vi "Change Macro Name in Listbox.vi"(9 "Call Data":variant, 10 "Popup Value":variant, 11 "Macros List in":cluster{"enabled?":bool, "macro name":string}[](array[cluster])) -> (3 "Macros List out":cluster{"enabled?":bool, "macro name":string}[](array[cluster]))   [LabVIEW 2016, in "Hardware.lvlib" / "Motions.lvlib" / "Motions Configuration.lvclass"]
uses:
  <userlib>/Common Components/Hardware/Abstract System/Motions/Motions Config/Motions Configuration.lvclass
  <userlib>/TSPopup/TSPopup.Grid.Cell Info.ctl
  <userlib>/TSPopup/TSPopup.Data Type.ctl
  <userlib>/TSPopup/TSPopup.lvclass
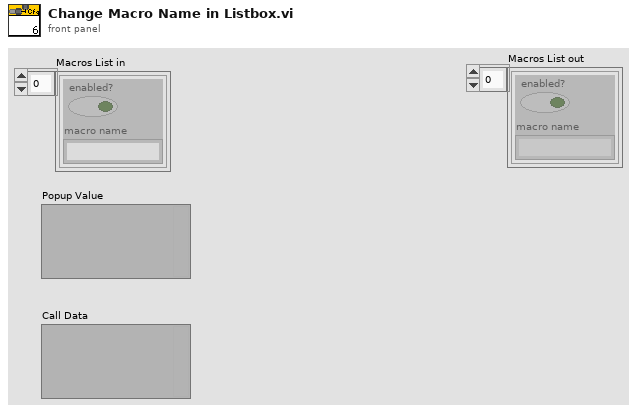
[diagram p1: front panel]
types:
  T1 = typedef "TSPopup.lvlib/TSPopup.lvclass/TSPopup.Grid.Cell Info.ctl" = cluster{"Tag":string, "Row":i32, "Column":i32, "In Symbol?":bool, "In Data?":bool, "Cell String":string, "Ctl Refnum":refnum<vi>, "Prop Type":T2, "Ring Strings":string[]}
  T2 = typedef "TSPopup.lvlib/TSPopup.lvclass/TSPopup.Data Type.ctl" = enum16{"Unkown", "NO POPUP", "String", "Integer", "Float", "Color", "Boolean", "Ring", "Captioned String", "Captioned Integer", "Button Color", "2 Int Cluster", "4 Int Cluster", "check"}
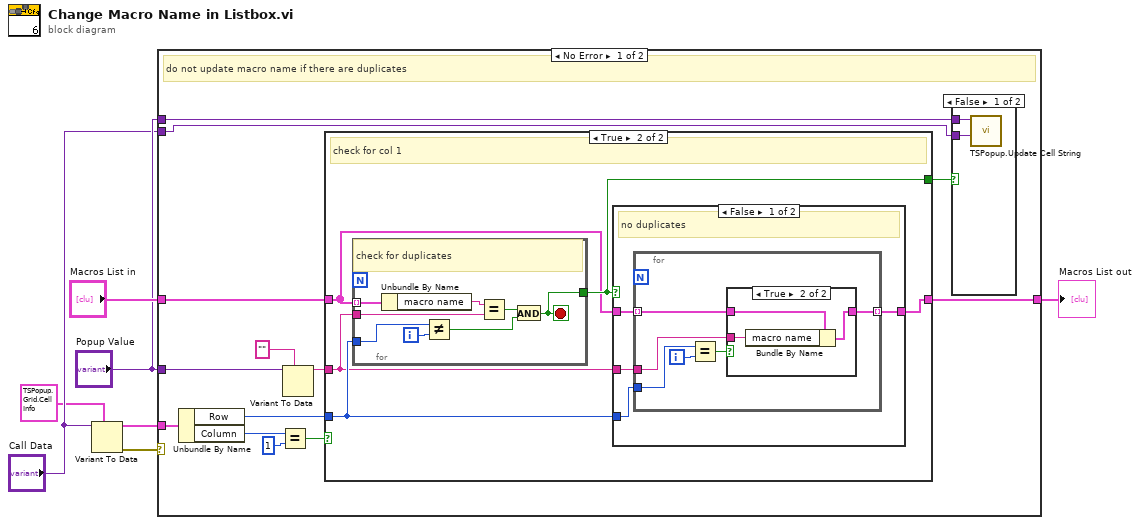
[diagram p0: block diagram]
diagram:
  n1 = Variant To Data(type=T1 {"Tag"="", "Row"=0, "Column"=0, "In Symbol?"=FALSE, "In Data?"=FALSE, "Cell String"="", "Ctl Refnum"=refnum, "Prop Type"=enum."Unkown", "Ring Strings"=[]} ("Cell Info (type only)"), Variant="Call Data") -> (data=w1:T1, error out=w2:errorcluster)  [unwired: 1 in]
  n2 = case shown="No Error" w2 {
    tunnel: w1 -> [w20 _]
    tunnel: "Popup Value" -> [w16 _]
    tunnel: "Macros List in" -> [w9 w52]
    tunnel: "Popup Value" -> [w11 _]
    tunnel: "Call Data" -> [w10 _]
    tunnel: [w8 w52] -> w7
    frame No Error {
      # "do not update macro name if there are duplicates"
      n3 = Unbundle By Name(w20) -> ("Row"=w14:i32, "Column"=w19:i32)
      n4 = Equal?(x=w19, y=1) -> (x = y?=w13:bool)
      n5 = Variant To Data(type="", Variant=w16) -> (data=w15:string)  [unwired: 1 in, 1 out]
      n6 = case shown="True" w13 {
        tunnel: w9 -> [w23 w27]
        tunnel: w15 -> [_ w25]
        tunnel: w14 -> [_ w26]
        tunnel: [_ w28] -> w12
        tunnel: [w23 w24] -> w8
        frame False {
        }
        frame True {
          # "check for col 1"
          n7 = for {
            tunnel: w27 -> [w51] mode=indexing
            tunnel: w25 -> [w50]
            tunnel: w26 -> [w48]
            tunnel: [w44] -> w28
            i -> [w47]
            stop <- w44 stop-if-true
            # "check for duplicates"
            n8 = Unbundle By Name(w51) -> ("macro name"=w49:string)
            n9 = Not Equal?(x=w48, y=w47) -> (x != y?=w45:bool)
            n10 = Equal?(x=w49, y=w50) -> (x = y?=w46:bool)
            n11 = And(x=w46, y=w45) -> (x .and. y?=w44:bool)
          }
          n12 = case shown="False" w28 {
            tunnel: w27 -> [w32 w43]
            tunnel: w26 -> [w31 _]
            tunnel: w25 -> [w30 _]
            tunnel: [w29 w43] -> w24
            frame False {
              # "no duplicates"
              n13 = for {
                tunnel: w32 -> [w36] mode=indexing
                tunnel: w31 -> [w37]
                tunnel: w30 -> [w35]
                tunnel: [w34] -> w29 mode=indexing
                i -> [w38]
                n14 = Equal?(x=w37, y=w38) -> (x = y?=w33:bool)
                n15 = case shown="True" w33 {
                  tunnel: w36 -> [w39 w42]
                  tunnel: w35 -> [_ w41]
                  tunnel: [w39 w40] -> w34
                  frame False {
                  }
                  frame True {
                    n16 = Bundle By Name(cluster=w42, "macro name"=w41) -> (w40:cluster{"enabled?":bool, "macro name":string})
                  }
                }
              }
            }
            frame True {
            }
          }
        }
      }
      n17 = case shown="False" w12 {
        tunnel: w11 -> [w22 _]
        tunnel: w10 -> [w21 _]
        frame False {
          n18 = call <userlib>:"TSPopup.Update Cell String.vi"("Call Data (must be Cell Info cluster)"=w21, "Popup Value"=w22) -> ()  [unwired: 9 in, 1 out]
        }
        frame True {
        }
      }
    }
    frame Error {
    }
  }
  "Macros List out" <- w7
